vi "Parameter Cluster to Array.vi"(11 "Parameter Cluster":T1) -> (3 "Array":dbl[](array[numeric]))   [LabVIEW 2020, in "Toggle 6.lvclass"]
doc: "This create an array from the parameter cluster.\nIf the parameter isn't enabled it returns an empty array.\nElse it returns an array of the values to sweep"
uses:
  Toggle 6.lvclass
  Controls/Parameter Cluster.ctl
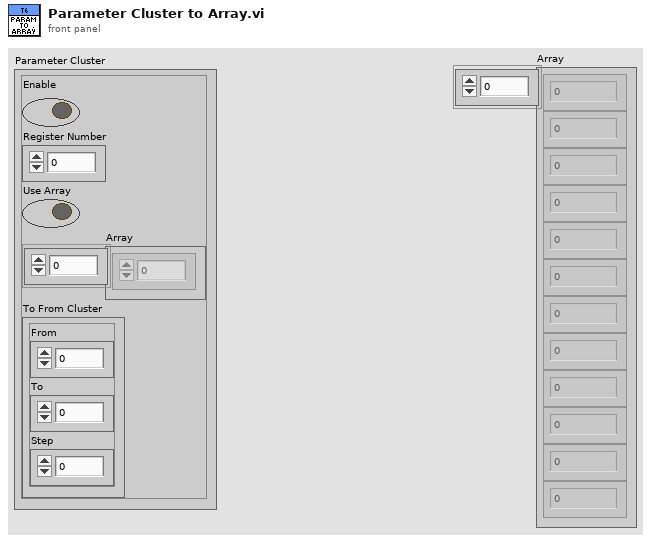
[diagram p1: front panel]
types:
  T1 = typedef "Toggle 6.lvclass/Parameter Cluster.ctl" = cluster{"Enable":bool, "Register Number":u32, "Use Array":bool, "Array":dbl[], "To From Cluster":cluster{"From":dbl, "To":dbl, "Step":dbl}}
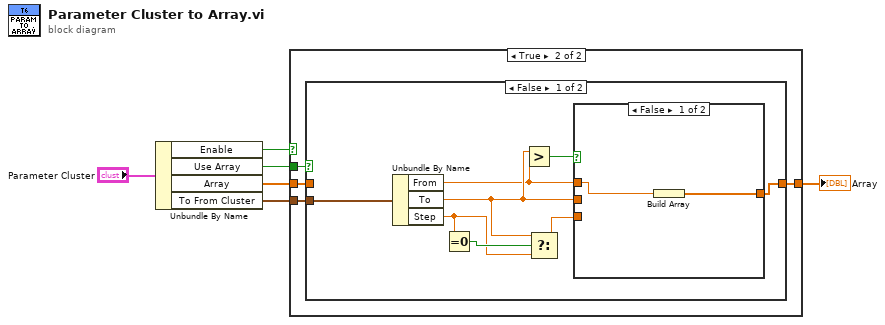
[diagram p0: block diagram]
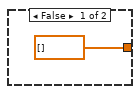
[diagram p2: hidden frame]
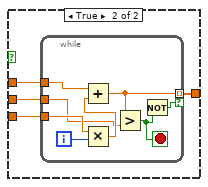
[diagram p3: hidden frame]
diagram:
  n1 = Unbundle By Name("Parameter Cluster") -> ("Enable"=w5:bool, "Use Array"=w4:bool, "Array"=w3:dbl[], "To From Cluster"=w2:cluster{"From":dbl, "To":dbl, "Step":dbl})
  n2 = case shown="True" w5 {
    tunnel: w4 -> [_ w11]
    tunnel: w3 -> [_ w10]
    tunnel: w2 -> [_ w9]
    tunnel: [dbl[] [] ("Array") w8] -> w1
    frame False {
    }
    frame True {
      n3 = case shown="False" w11 {
        tunnel: w10 -> [_ w34]
        tunnel: w9 -> [w19 _]
        tunnel: [w18 w34] -> w8
        frame False {
          n4 = Unbundle By Name(w19) -> ("From"=w13:dbl, "To"=w14:dbl, "Step"=w16:dbl)
          n5 = Equal To 0?(x=w16) -> (x = 0?=w17:bool)
          n6 = Greater?(x=w14, y=w13) -> (0:w12:bool)
          n7 = Select(t=w14, s=w17, f=w16) -> (s? t:f=w15:dbl)
          n8 = case shown="False" w12 {
            tunnel: [w20 w25] -> w18
            tunnel: w15 -> [_ w24]
            tunnel: w14 -> [_ w23]
            tunnel: w13 -> [w21 w22]
            frame False {
              n9 = Build Array(w21) -> (w20:dbl[])
            }
            frame True {
              n10 = while {
                tunnel: w23 -> [w28]
                tunnel: w24 -> [w31]
                tunnel: [w29] -> w25 mode=indexing if=w27
                tunnel: w22 -> [w33]
                i -> [w32]
                stop <- w26 stop-if-true
                n11 = Multiply(x=w31, y=w32) -> (x*y=w30:dbl)
                n12 = Add(x=w33, y=w30) -> (x+y=w29:dbl)
                n13 = Greater?(x=w29, y=w28) -> (0:w26:bool)
                n14 = Not(x=w26) -> (.not. x?=w27:bool)
              }
            }
          }
        }
        frame True {
        }
      }
    }
  }
  "Array" <- w1
